vi "Test Class Name.vi"() -> ()   [LabVIEW 2014]
uses:
  PPT/PPT.lvclass
  <vilib>/regexp/Match Regular Expression.xnode
panel:
  out "substring before match":string
  out "class name 2":string
  out "before match":string
  out "class name":string
  out "after substring":string
  out "before substring":string
  out "offset past match":i32
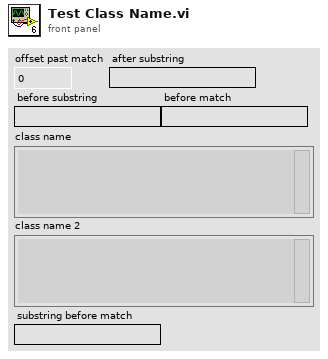
[diagram p1: front panel]
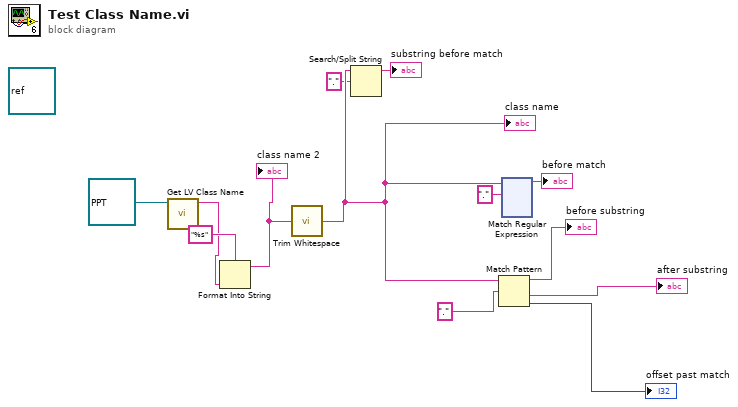
[diagram p0: block diagram]
diagram:
  (unwired) refnum<class> refnum ("LabVIEW Object")
  n1 = call <vilib>:"Get LV Class Name.vi"("object"=refnum<class "PPT.lvclass"> refnum ("PPT")) -> ("class name"=w4:string)  [unwired: 9 in, 1 out]
  n2 = Format Into String(format string="%s", w4) -> (resulting string=w5:string)  [unwired: 2 in, 1 out]
  "class name 2" <- w5
  n3 = call <vilib>:"Trim Whitespace.vi"("string"=w5) -> ("trimmed string"=w3:string)  [unwired: 1 in]
  "class name" <- w3
  n4 = Search/Split String(string=w3, search string/char (-)=".") -> (substring before match=→"substring before match":string)  [unwired: 1 in, 2 out]
  n5 = Match Pattern(string=w3, regular expression=".") -> (before substring=→"before substring":string, after substring=→"after substring":string, offset past match=→"offset past match":i32)  [unwired: 1 in, 1 out]
  n6 = xnode "Match Regular Expression"("input string"=w3, "regular expression"=".") -> ("before match"=→"before match":string)  [unwired: 4 in, 4 out]
